vi "executeOffensivePlay.vi"(8 "error in (no error)":errorcluster, 11 "Game in":refnum<class "Game.lvclass">) -> (0 "error out":errorcluster, 3 "Game out":refnum<class "Game.lvclass">)   [LabVIEW 2023, in "Game.lvclass"]
uses:
  Game.lvclass
  Utilities_class/Utilities.lvclass
  Team_class/OffensivePlay.ctl
  Game.lvclass/Game.ctl
  Team_class/Team.lvclass/Team.ctl
  Playbook_class/Playbook.lvclass/Playbook.ctl
  TestPlay_class/TestPlay.lvclass/TestPlay.ctl
  EnemyPossessionAtOurFieldPlay_class/EnemyPossessionAtOurFieldPlay.lvclass/EnemyPossessionAtOurFieldPlay.ctl
  PreparePassPlay_class/PreparePassPlay.lvclass/PreparePassPlay.ctl
  PrepareDoublePassPlay_class/PrepareDoublePassPlay.lvclass/PrepareDoublePassPlay.ctl
  PrepareRollToPassPlay_class/PrepareRollToPassPlay.lvclass/PrepareRollToPassPlay.ctl
  TableWithStrikerPlay_class/TableWithStrikerPlay.lvclass/TableWithStrikerPlay.ctl
  TableWith2ndStrikerPlay_class/TableWith2ndStrikerPlay.lvclass/TableWith2ndStrikerPlay.ctl
  DirectEnemyPlay_class/DirectEnemyPlay.lvclass/DirectEnemyPlay.ctl
  HaltPlay_class/HaltPlay.lvclass/HaltPlay.ctl
  IndirectEnemyPlay_class/IndirectEnemyPlay.lvclass/IndirectEnemyPlay.ctl
  StopOffensivePlay_class/StopOffensivePlay.lvclass/StopOffensivePlay.ctl
  BallOutOfFieldPlay_class/BallOutOfFieldPlay.lvclass/BallOutOfFieldPlay.ctl
  EnemyPossessionAtEnemyFieldPlay_class/EnemyPossessionAtEnemyFieldPlay.lvclass/EnemyPossessionAtEnemyFieldPlay.ctl
  NormalGamePlay_class/NormalGamePlay.lvclass/NormalGamePlay.ctl
  PrepareKickoffAllyPlay_class/PrepareKickoffAllyPlay.lvclass/PrepareKickoffAllyPlay.ctl
  PreparePenaltyAllyPlay_class/PreparePenaltyAllyPlay.lvclass/PreparePenaltyAllyPlay.ctl
  PreparePenaltyEnemyPlay_class/PreparePenaltyEnemyPlay.lvclass/PreparePenaltyEnemyPlay.ctl
  PrepareKickoffEnemyPlay_class/PrepareKickoffEnemyPlay.lvclass/PrepareKickoffEnemyPlay.ctl
  KickPenaltyAllyPlay_class/KickPenaltyAllyPlay.lvclass/KickPenaltyAllyPlay.ctl
  Robot_class/Robot.lvclass/Robot.ctl
  PreparePassReceiverRole_class/PreparePassReceiverEnum.ctl
  Robot_class/Read role.vi
  Playbook_class/Read offensive_plays.vi
  TestPlay_class/Read Roles.vi
  EnemyPossessionAtOurFieldPlay_class/Read Roles.vi
  PreparePassPlay_class/Read Roles.vi
  PrepareDoublePassPlay_class/Read Roles.vi
  PrepareRollToPassPlay_class/Read Roles.vi
  TableWithStrikerPlay_class/Read Roles.vi
  TableWith2ndStrikerPlay_class/Read Roles.vi
  DirectEnemyPlay_class/Read Roles.vi
  HaltPlay_class/Read Roles.vi
  IndirectEnemyPlay_class/Read Roles.vi
  StopOffensivePlay_class/Read Roles.vi
  BallOutOfFieldPlay_class/Read Roles.vi
  EnemyPossessionAtEnemyFieldPlay_class/Read Roles.vi
  NormalGamePlay_class/Read Roles.vi
  PrepareKickoffAllyPlay_class/Read Roles.vi
  PreparePenaltyAllyPlay_class/Read Roles.vi
  Robot_class/Read id.vi
  PreparePenaltyEnemyPlay_class/Read roles.vi
  PrepareKickoffEnemyPlay_class/Read Roles.vi
  KickPenaltyAllyPlay_class/Read Roles.vi
  Read OffensiveTeam.vi
  Team_class/Read RobotRef.vi
  Team_class/Read OffensivePlay.vi
  Team_class/Write RobotRef.vi
  Team_class/Write OffensivePlay Finished.vi
  Write OffensiveTeam.vi
  Ally_class/Ally.lvclass
  C:/Users/roboi/Downloads/VSS_AI-Larc2023/Team_class/Team.lvclass
  Playbook_class/Playbook.lvclass
  Robot_class/Robot.lvclass
  Play_class/Play.lvclass
  TestPlay_class/TestPlay.lvclass
  EnemyPossessionAtEnemyFieldPlay_class/EnemyPossessionAtEnemyFieldPlay.lvclass
  EnemyPossessionAtOurFieldPlay_class/EnemyPossessionAtOurFieldPlay.lvclass
  NormalGamePlay_class/NormalGamePlay.lvclass
  IndirectEnemyPlay_class/IndirectEnemyPlay.lvclass
  PrepareKickoffAllyPlay_class/PrepareKickoffAllyPlay.lvclass
  PrepareKickoffEnemyPlay_class/PrepareKickoffEnemyPlay.lvclass
  KickPenaltyAllyPlay_class/KickPenaltyAllyPlay.lvclass
  PreparePenaltyAllyPlay_class/PreparePenaltyAllyPlay.lvclass
  DirectEnemyPlay_class/DirectEnemyPlay.lvclass
  PreparePenaltyEnemyPlay_class/PreparePenaltyEnemyPlay.lvclass
  BallOutOfFieldPlay_class/BallOutOfFieldPlay.lvclass
  StopOffensivePlay_class/StopOffensivePlay.lvclass
  PassPlay_class/PassPlay.lvclass
  DirectKickPlay_class/DirectKickPlay.lvclass
  HaltPlay_class/HaltPlay.lvclass
  PreparePassPlay_class/PreparePassPlay.lvclass
  PassToStriker_class/PassToStriker.lvclass
  PassTo2ndStriker_class/PassTo2ndStriker.lvclass
  SimplePass_class/SimplePass.lvclass
  PrepareRollToPassPlay_class/PrepareRollToPassPlay.lvclass
  PrepareDoublePassPlay_class/PrepareDoublePassPlay.lvclass
  TableWith2ndStrikerPlay_class/TableWith2ndStrikerPlay.lvclass
  TableWithStrikerPlay_class/TableWithStrikerPlay.lvclass
  TestRole_class/TestRole.lvclass
  Role_class/Role.lvclass
  ShootRole_class/ShootRole.lvclass
  MarkerRole_class/MarkerRole.lvclass
  PreparePassReceiverRole_class/PreparePassReceiverRole.lvclass
  AttackerStopRole_class/AttackerStopRole.lvclass
  PrepareRollToPassReceiverRole_class/PrepareRollToPassReceiverRole.lvclass
  PrepareRollToPassRollerRole_class/PrepareRollToPassRollerRole.lvclass
  PassKickerRole_class/PassKickerRole.lvclass
  PassReceiverRole_class/PassReceiverRole.lvclass
  PassObserverRole_class/PassObserverRole.lvclass
  TableFinalizerRole_class/TableFinalizerRole.lvclass
  TablerRole_class/TablerRole.lvclass
  AttackerBlockRole_class/AttackerBlockRole.lvclass
  HaltRole_class/HaltRole.lvclass
  BallOutOfFieldRole_class/BallOutOfFieldRole.lvclass
  FollowAttackerRole_class/FollowAttackerRole.lvclass
  AttackerAimGoalRole_class/AttackerAimGoalRole.lvclass
  PenaltyDefenseRole_class/PenaltyDefenseRole.lvclass
  SimplePassRollRole_class/SimplePassRollRole.lvclass
  SimplePassReceiverRole_class/SimplePassReceiverRole.lvclass
  PenaltyAttackerRole_class/PenaltyAttackerRole.lvclass
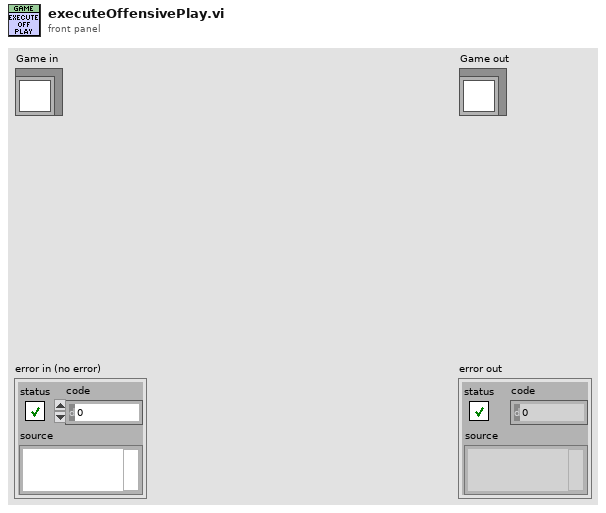
[diagram p1: front panel]
types:
  T1 = typedef "OffensivePlay.ctl" = enum16{"TableWithStriker", "TableWith2ndStrikerPlay", "PrepareDoublePass", "PrepareRollToPass", "SimplePass", "PreparePass", "PassToStriker", "BallOutOfField", "PassTo2ndStriker", "StopOffensive", "Prepare Penalty Enemy", "EnemyPossessionAtEnemyField", "EnemyPossesionAtOurField", "TestPlay", "PreparePenaltyAlly", "KickPenaltyAlly", "PrepareKickoffAlly", "PrepareKickoffEnemy", "IndirectEnemy", "DirectEnemy", "NormalGame", "DirectKick", "Pass", "Halt", "Timeout", "PassPlay", "PenaltyEnemy"}
  T2 = typedef "PreparePassReceiverEnum.ctl" = enum16{"2ndStrikerDPass", "2ndStriker", "Striker"}
  T3 = typedef "offensive_plays.ctl" = cluster{"Play":refnum<class "Play.lvclass">, "TestPlay":refnum<class "TestPlay.lvclass">, "EnemyPossessionAtEnemyFieldPlay":refnum<class "EnemyPossessionAtEnemyFieldPlay.lvclass">, "EnemyPossessionAtOurFieldPlay":refnum<class "EnemyPossessionAtOurFieldPlay.lvclass">, "NormalGamePlay":refnum<class "NormalGamePlay.lvclass">, "IndirectEnemyPlay":refnum<class "IndirectEnemyPlay.lvclass">, "PrepareKickoffAllyPlay":refnum<class "PrepareKickoffAllyPlay.lvclass">, "PrepareKickoffEnemyPlay":refnum<class "PrepareKickoffEnemyPlay.lvclass">, "KickPenaltyAllyPlay":refnum<class "KickPenaltyAllyPlay.lvclass">, "PreparePenaltyAllyPlay":refnum<class "PreparePenaltyAllyPlay.lvclass">, "DirectEnemyPlay":refnum<class "DirectEnemyPlay.lvclass">, "PreparePenaltyEnemyPlay":refnum<class "PreparePenaltyEnemyPlay.lvclass">, "BallOutOfFieldPlay":refnum<class "BallOutOfFieldPlay.lvclass">, "StopOffensivePlay":refnum<class "StopOffensivePlay.lvclass">, "PassPlay":refnum<class "PassPlay.lvclass">, "DirectKickPlay":refnum<class "DirectKickPlay.lvclass">, "HaltPlay":refnum<class "HaltPlay.lvclass">, "PreparePassPlay":refnum<class "PreparePassPlay.lvclass">, "PassToStrikerPlay":refnum<class "PassToStriker.lvclass">, "PassTo2ndStrikerPlay":refnum<class "PassTo2ndStriker.lvclass">, "SimplePassPlay":refnum<class "SimplePass.lvclass">, "PrepareRollToPassPlay":refnum<class "PrepareRollToPassPlay.lvclass">, "PrepareDoublePassPlay":refnum<class "PrepareDoublePassPlay.lvclass">, "TableWith2ndStrikerPlay":refnum<class "TableWith2ndStrikerPlay.lvclass">, "TableWithStrikerPlay":refnum<class "TableWithStrikerPlay.lvclass">}
  T4 = typedef "roles.ctl" = enum16{"BallChallengerAttackerVSS", "NormalAttackerVSS", "AttackerAimGoalVSS", "DefenderAreaVSS", "KeeperVSS", "Tabler", "TableFinalizer", "PrepareRollToPassRoller", "PrepareRollToPassReceiver", "SimplePassRoll", "SimplePassRollReceiver", "PenaltyDefense", "PreparePassReceiver 2", "PreparePassReceiver 1", "PassObserver", "Timeout", "Goto", "ZigZag", "None", "BallOutOfField", "DefenderArea", "Duelist", "AttackerStop", "FollowAttacker", "KeeperRole", "KickPenalty", "AttackerAimGoal", "AttackerBlock", "Marker", "Halt", "Shoot", "PassKicker", "PassReceiver", "TestRole", "PenaltyAttacker"}
  T5 = cluster{"TestRole 1":refnum<class "TestRole.lvclass">, "Role":refnum<class "Role.lvclass">, "TestRole 2":refnum<class "TestRole.lvclass">, "TestRole 3":refnum<class "TestRole.lvclass">}
  T6 = cluster{"ShootRole":refnum<class "ShootRole.lvclass">, "MarkerRole":refnum<class "MarkerRole.lvclass">}
  T7 = cluster{"PreparePassReceiverRole 1":refnum<class "PreparePassReceiverRole.lvclass">, "AttackerStopRole":refnum<class "AttackerStopRole.lvclass">, "PreparePassReceiverRole 2":refnum<class "PreparePassReceiverRole.lvclass">}
  T8 = cluster{"AttackerStopRole":refnum<class "AttackerStopRole.lvclass">, "PreparePassReceiverRole 1":refnum<class "PreparePassReceiverRole.lvclass">, "PreparePassReceiverRole 2":refnum<class "PreparePassReceiverRole.lvclass">}
  T9 = cluster{"PreparePassReceiverRole 1":refnum<class "PreparePassReceiverRole.lvclass">, "PreparePassReceiverRole 2":refnum<class "PreparePassReceiverRole.lvclass">, "PrepareRollToPassReceiverRole":refnum<class "PrepareRollToPassReceiverRole.lvclass">, "PrepareRollToPassRollerRole":refnum<class "PrepareRollToPassRollerRole.lvclass">}
  T10 = cluster{"PassKickerRole":refnum<class "PassKickerRole.lvclass">, "PassReceiverRole":refnum<class "PassReceiverRole.lvclass">, "PassObserverRole":refnum<class "PassObserverRole.lvclass">}
  T11 = cluster{"TableFinalizerRole":refnum<class "TableFinalizerRole.lvclass">, "TablerRole":refnum<class "TablerRole.lvclass">, "PassObserverRole":refnum<class "PassObserverRole.lvclass">}
  T12 = cluster{"AttackerBlockRole":refnum<class "AttackerBlockRole.lvclass">, "MarkerRole":refnum<class "MarkerRole.lvclass">}
  T13 = cluster{"HaltRole 1":refnum<class "HaltRole.lvclass">, "HaltRole 2":refnum<class "HaltRole.lvclass">, "HaltRole 3":refnum<class "HaltRole.lvclass">, "HaltRole 4":refnum<class "HaltRole.lvclass">, "HaltRole 5":refnum<class "HaltRole.lvclass">, "HaltRole 6":refnum<class "HaltRole.lvclass">}
  T14 = cluster{"MarkerRole":refnum<class "MarkerRole.lvclass">, "AttackerStopRole":refnum<class "AttackerStopRole.lvclass">}
  T15 = cluster{"BallOutOfFieldRole":refnum<class "BallOutOfFieldRole.lvclass">, "FollowAttackerRole":refnum<class "FollowAttackerRole.lvclass">}
  T16 = cluster{"ShootRole":refnum<class "ShootRole.lvclass">, "FollowAttackerRole":refnum<class "FollowAttackerRole.lvclass">}
  T17 = cluster{"AttackerAimGoalRole":refnum<class "AttackerAimGoalRole.lvclass">, "FollowAttackerRole":refnum<class "FollowAttackerRole.lvclass">}
  T18 = cluster{"AttackerAimGoalRole":refnum<class "AttackerAimGoalRole.lvclass">}
  T19 = cluster{"PenaltyDefenseRole 1":refnum<class "PenaltyDefenseRole.lvclass">, "PenaltyDefenseRole 2":refnum<class "PenaltyDefenseRole.lvclass">, "PenaltyDefenseRole 3":refnum<class "PenaltyDefenseRole.lvclass">, "PenaltyDefenseRole 4":refnum<class "PenaltyDefenseRole.lvclass">, "PenaltyDefenseRole 5":refnum<class "PenaltyDefenseRole.lvclass">}
  T20 = cluster{"SimplePassRollRole":refnum<class "SimplePassRollRole.lvclass">, "SimplePassReceiverRole":refnum<class "SimplePassReceiverRole.lvclass">}
  T21 = cluster{"AttackerBlockRole":refnum<class "AttackerBlockRole.lvclass">, "FollowAttackerRole":refnum<class "FollowAttackerRole.lvclass">}
  T22 = cluster{"PenaltyAttackerRole":refnum<class "PenaltyAttackerRole.lvclass">}
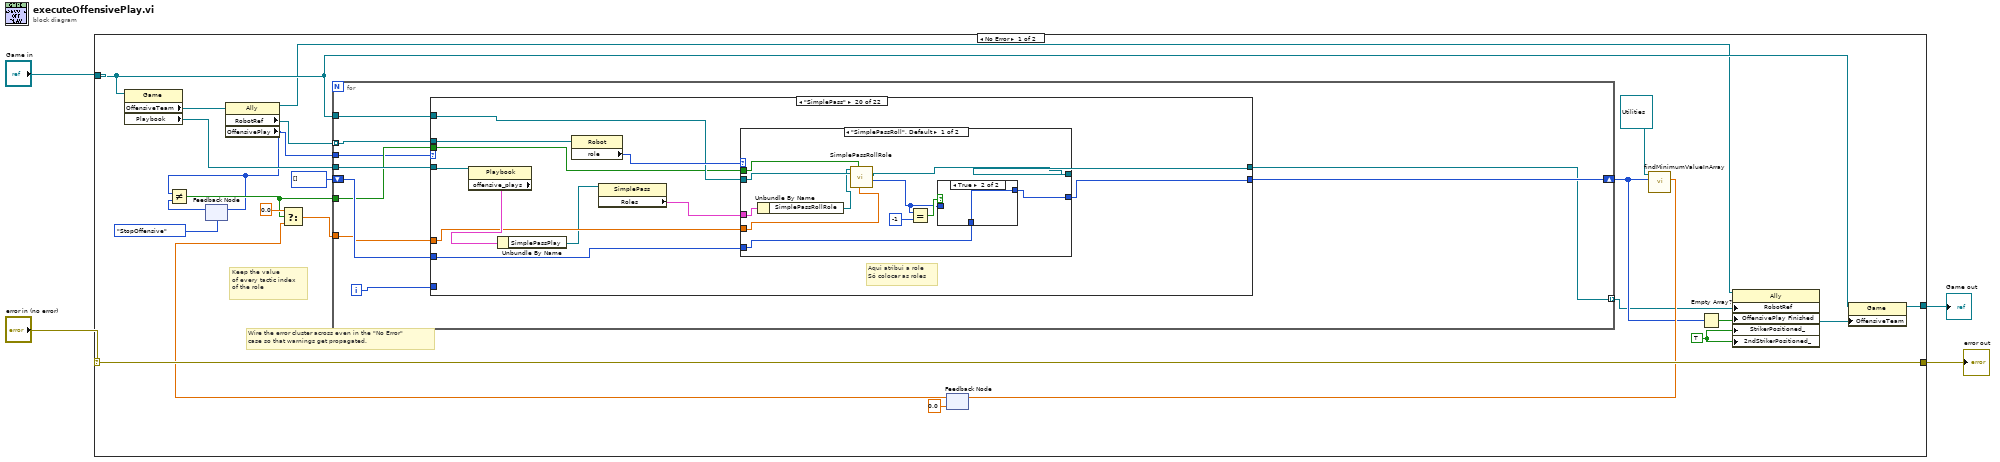
[diagram p0: block diagram]
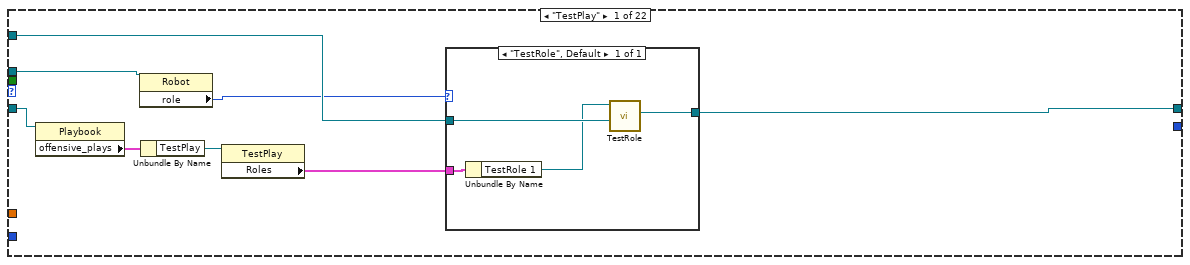
[diagram p2: hidden frame]
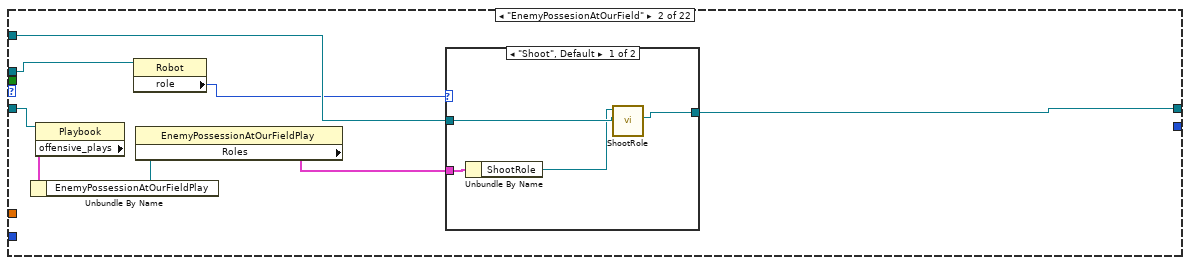
[diagram p3: hidden frame]
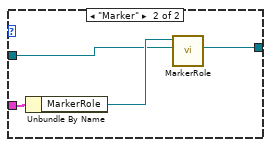
[diagram p4: hidden frame]
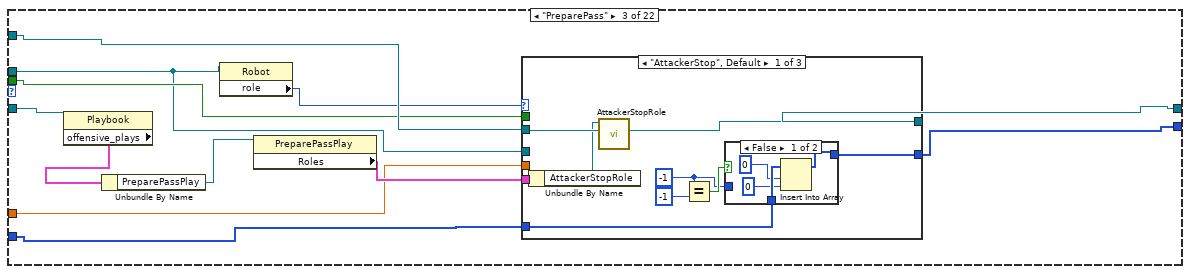
[diagram p5: hidden frame]
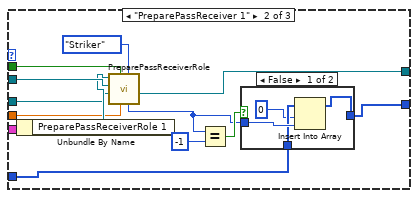
[diagram p7: hidden frame]
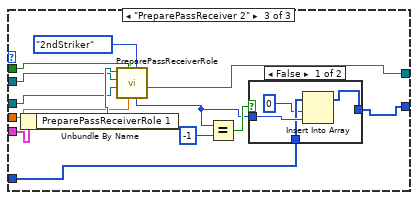
[diagram p9: hidden frame]
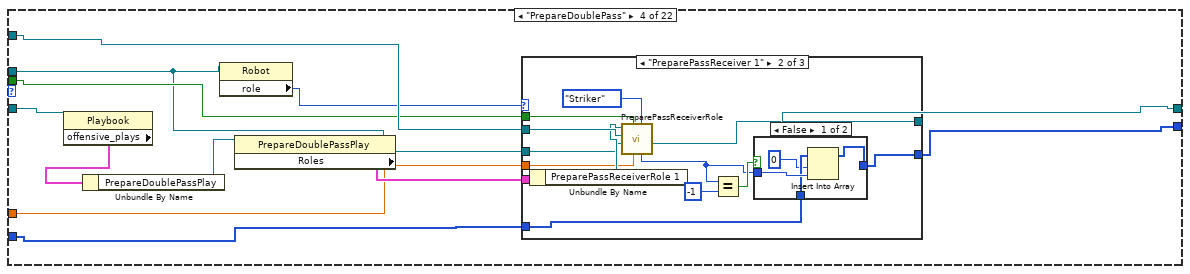
[diagram p11: hidden frame]
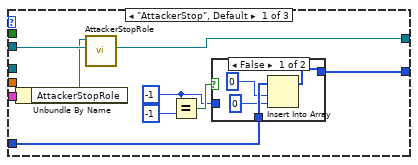
[diagram p12: hidden frame]
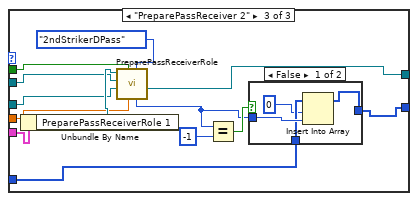
[diagram p15: hidden frame]
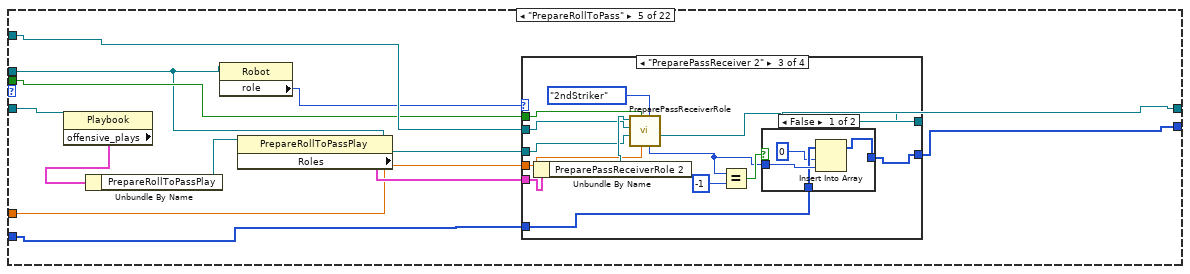
[diagram p17: hidden frame]
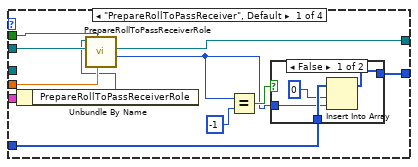
[diagram p18: hidden frame]
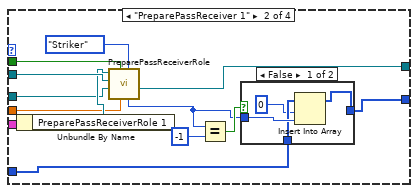
[diagram p20: hidden frame]
diagram:
  n1 = case shown="No Error" "error in (no error)" {
    selector: "error in (no error)" -> [w27 w748]
    tunnel: [w27 w748] -> w1
    tunnel: [w23 w747] -> w2
    tunnel: "Game in" -> [w8 w747]
    frame No Error {
      w10 = TRUE
      # "Keep the value\nof every tactic index\nof the role"
      # "Wire the error cluster across even in the \"No Error\"\ncase so that warnings get propagated."
      n2 = property class="Game"(reference=w8) -> ("OffensiveTeam"=w26:refnum<class "Ally.lvclass">, "Playbook"=w24:refnum<class "Playbook.lvclass">)  [unwired: 1 in, 2 out]
      n3 = feedback #1(OffensivePlay."StopOffensive" ("OffensivePlay")) -> (w18:T1)
      n4 = property class="Ally"(reference=w26) -> (reference out=w7:refnum<class "Ally.lvclass">, "RobotRef"=w25:refnum<class "Robot.lvclass">[], "OffensivePlay"=w5:T1)  [unwired: 1 in, 1 out]
      n5 = Not Equal?(x=w5, y=w18) -> (x != y?=w14:bool)
      n6 = feedback-in #1(w5) -> ()
      n7 = feedback #2(0.0 ("minimum")) -> (w16:dbl)
      n8 = Select(t=0.0, s=w14, f=w16) -> (s? t:f=w9:dbl)
      n9 = for {
        tunnel: w25 -> [w32] mode=indexing
        tunnel: w24 -> [w37]
        tunnel: w8 -> [w36]
        shift-right: [w35] -> w12
        shift-left: i32[] [] -> [w34]
        tunnel: w14 -> [w33]
        tunnel: w9 -> [w31]
        tunnel: [w29] -> w6 mode=indexing
        tunnel: w5 -> [w28]
        i -> [w30]
        n10 = case shown="\"SimplePass\"" w28 {
          tunnel: w37 -> [w45 w57 w70 w132 w194 w277 w337 w397 w457 w517 w533 w545 w561 w577 w593 w609 w625 w641 w654 w680 w726 w742]
          tunnel: w36 -> [w41 w53 w72 w134 w196 w279 w340 w400 w460 w513 w529 w541 w557 w573 w589 w605 w621 w637 w650 w682 w722 w738]
          tunnel: [w40 w52 w75 w137 w199 w274 w336 w396 w456 w512 w528 w540 w556 w572 w588 w604 w620 w636 w648 w684 w721 w737] -> w29
          tunnel: w31 -> [_ _ w68 w130 w192 w270 w330 w390 w450 _ _ _ _ _ _ _ _ _ _ w679 _ _]
          tunnel: [_ _ w74 w136 w198 w273 w335 w395 w455 _ _ _ _ _ _ _ _ _ _ w683 _ _] -> w35
          tunnel: w34 -> [_ _ w73 w135 w197 w272 w334 w394 w454 _ _ _ _ _ _ _ _ _ _ w678 _ _]
          tunnel: w33 -> [_ _ w71 w133 w195 w271 w338 w398 w458 _ _ _ _ _ _ _ _ _ _ w681 _ _]
          tunnel: w32 -> [w39 w51 w67 w129 w191 w278 w339 w399 w459 w511 w527 w539 w554 w571 w587 w603 w619 w635 w649 w677 w720 w736]
          tunnel: w30 -> [_ _ _ _ _ _ _ _ _ _ _ _ _ _ _ _ _ _ w646 _ _ _]
          frame "TestPlay" {
            n11 = property class="Playbook"(reference=w45) -> ("offensive_plays"=w44:T3)  [unwired: 1 in, 2 out]
            n12 = property class="Robot"(reference=w39) -> ("role"=w38:T4)  [unwired: 1 in, 2 out]
            n13 = Unbundle By Name(w44) -> ("TestPlay"=w43:refnum<class "TestPlay.lvclass">)
            n14 = property class="TestPlay"(reference=w43) -> ("Roles"=w42:T5)  [unwired: 1 in, 2 out]
            n15 = case shown="\"TestRole\", Default" w38 {
              tunnel: w42 -> [w49]
              tunnel: w41 -> [w48]
              tunnel: [w47] -> w40
              frame "TestRole", Default {
                n16 = Unbundle By Name(w49) -> ("TestRole 1"=w46:refnum<class "TestRole.lvclass">)
                n17 = call-dynamic "TestRole.vi"("Game in"=w48, "TestRole in"=w46) -> ("Robot out"=w47:refnum<class "Robot.lvclass">)  [unwired: 6 in, 3 out]
              }
            }
          }
          frame "EnemyPossesionAtOurField" {
            n18 = property class="Playbook"(reference=w57) -> ("offensive_plays"=w56:T3)  [unwired: 1 in, 2 out]
            n19 = Unbundle By Name(w56) -> ("EnemyPossessionAtOurFieldPlay"=w55:refnum<class "EnemyPossessionAtOurFieldPlay.lvclass">)
            n20 = property class="Robot"(reference=w51) -> ("role"=w50:T4)  [unwired: 1 in, 2 out]
            n21 = property class="EnemyPossessionAtOurFieldPlay"(reference=w55) -> ("Roles"=w54:T6)  [unwired: 1 in, 2 out]
            n22 = case shown="\"Shoot\", Default" w50 {
              tunnel: w54 -> [w61 w65]
              tunnel: w53 -> [w60 w63]
              tunnel: [w58 w62] -> w52
              frame "Shoot", Default {
                n23 = Unbundle By Name(w61) -> ("ShootRole"=w59:refnum<class "ShootRole.lvclass">)
                n24 = call-dynamic "ShootRole.vi"("Game in"=w60, "ShootRole in"=w59) -> ("Robot out"=w58:refnum<class "Robot.lvclass">)  [unwired: 6 in, 3 out]
              }
              frame "Marker" {
                n25 = Unbundle By Name(w65) -> ("MarkerRole"=w64:refnum<class "MarkerRole.lvclass">)
                n26 = call-dynamic "MarkerRole.vi"("Game in"=w63, "MarkerRole in"=w64) -> ("Robot out"=w62:refnum<class "Robot.lvclass">)  [unwired: 6 in, 3 out]
              }
            }
          }
          frame "PreparePass" {
            n27 = property class="Playbook"(reference=w70) -> ("offensive_plays"=w69:T3)  [unwired: 1 in, 2 out]
            n28 = Unbundle By Name(w69) -> ("PreparePassPlay"=w76:refnum<class "PreparePassPlay.lvclass">)
            n29 = property class="Robot"(reference=w67) -> ("role"=w66:T4)  [unwired: 1 in, 2 out]
            n30 = property class="PreparePassPlay"(reference=w76) -> ("Roles"=w77:T7)  [unwired: 1 in, 2 out]
            n31 = case shown="\"AttackerStop\", Default" w66 {
              tunnel: w77 -> [w86 w101 w118]
              tunnel: w72 -> [w81 w102 w113]
              tunnel: [w85 w97 w115] -> w75
              tunnel: [w83 w96 w116] -> w74
              tunnel: w73 -> [w82 w99 w117]
              tunnel: w71 -> [_ w95 w114]
              tunnel: w68 -> [_ w94 w111]
              tunnel: w67 -> [_ w93 w112]
              frame "AttackerStop", Default {
                w78 = -1 ("x")
                n32 = Unbundle By Name(w86) -> ("AttackerStopRole"=w80:refnum<class "AttackerStopRole.lvclass">)
                n33 = call-dynamic "AttackerStopRole.vi"("Game in"=w81, "AttackerStopRole in"=w80) -> ("Robot out"=w85:refnum<class "Robot.lvclass">)  [unwired: 6 in, 3 out]
                n34 = Equal?(x=w78, y=-1) -> (x = y?=w84:bool)
                n35 = case shown="False" w84 {
                  tunnel: w82 -> [w90 w91]
                  tunnel: [w89 w91] -> w83
                  tunnel: w78 -> [_ _]
                  frame False {
                    n36 = Insert Into Array(array=w90, index=0, new element=0 ("new element/subarray")) -> (w89:i32[])
                  }
                  frame True {
                  }
                }
              }
              frame "PreparePassReceiver 1" {
                n37 = Unbundle By Name(w101) -> ("PreparePassReceiverRole 1"=w100:refnum<class "PreparePassReceiverRole.lvclass">)
                n38 = call "PreparePassReceiverRole.vi"("Striker/2ndStriker"=PreparePassReceiverEnum."Striker", "Tactic index in"=w94, "first call"=w95, "RobotRef"=w93, "Game in"=w102, "PreparePassReceiverRole in"=w100) -> ("Robot out"=w97:refnum<class "Robot.lvclass">, "tactic index"=w98:i32)  [unwired: 1 in, 3 out]
                n39 = Equal?(x=w98, y=-1) -> (x = y?=w103:bool)
                n40 = case shown="False" w103 {
                  tunnel: w98 -> [w108 _]
                  tunnel: w99 -> [w107 w109]
                  tunnel: [w105 w109] -> w96
                  frame False {
                    n41 = Insert Into Array(array=w107, index=0, new element=w108) -> (w105:i32[])
                  }
                  frame True {
                  }
                }
              }
              frame "PreparePassReceiver 2" {
                n42 = Unbundle By Name(w118) -> ("PreparePassReceiverRole 1"=w120:refnum<class "PreparePassReceiverRole.lvclass">)
                n43 = call "PreparePassReceiverRole.vi"("Striker/2ndStriker"=PreparePassReceiverEnum."2ndStriker", "Tactic index in"=w111, "first call"=w114, "RobotRef"=w112, "Game in"=w113, "PreparePassReceiverRole in"=w120) -> ("Robot out"=w115:refnum<class "Robot.lvclass">, "tactic index"=w119:i32)  [unwired: 1 in, 3 out]
                n44 = Equal?(x=w119, y=-1) -> (x = y?=w121:bool)
                n45 = case shown="False" w121 {
                  tunnel: w119 -> [w126 _]
                  tunnel: w117 -> [w125 w127]
                  tunnel: [w123 w127] -> w116
                  frame False {
                    n46 = Insert Into Array(array=w125, index=0, new element=w126) -> (w123:i32[])
                  }
                  frame True {
                  }
                }
              }
            }
          }
          frame "PrepareDoublePass" {
            n47 = property class="Playbook"(reference=w132) -> ("offensive_plays"=w131:T3)  [unwired: 1 in, 2 out]
            n48 = Unbundle By Name(w131) -> ("PrepareDoublePassPlay"=w138:refnum<class "PrepareDoublePassPlay.lvclass">)
            n49 = property class="Robot"(reference=w129) -> ("role"=w128:T4)  [unwired: 1 in, 2 out]
            n50 = property class="PrepareDoublePassPlay"(reference=w138) -> ("Roles"=w139:T8)  [unwired: 1 in, 2 out]
            n51 = case shown="\"PreparePassReceiver 1\"" w128 {
              tunnel: w139 -> [w148 w163 w180]
              tunnel: w134 -> [w143 w164 w175]
              tunnel: [w147 w159 w177] -> w137
              tunnel: [w145 w158 w178] -> w136
              tunnel: w135 -> [w144 w161 w179]
              tunnel: w133 -> [_ w157 w176]
              tunnel: w130 -> [_ w156 w173]
              tunnel: w129 -> [_ w155 w174]
              frame "AttackerStop", Default {
                w140 = -1 ("x")
                n52 = Unbundle By Name(w148) -> ("AttackerStopRole"=w142:refnum<class "AttackerStopRole.lvclass">)
                n53 = call-dynamic "AttackerStopRole.vi"("Game in"=w143, "AttackerStopRole in"=w142) -> ("Robot out"=w147:refnum<class "Robot.lvclass">)  [unwired: 6 in, 3 out]
                n54 = Equal?(x=w140, y=-1) -> (x = y?=w146:bool)
                n55 = case shown="False" w146 {
                  tunnel: w144 -> [w152 w153]
                  tunnel: [w151 w153] -> w145
                  tunnel: w140 -> [_ _]
                  frame False {
                    n56 = Insert Into Array(array=w152, index=0, new element=0 ("new element/subarray")) -> (w151:i32[])
                  }
                  frame True {
                  }
                }
              }
              frame "PreparePassReceiver 1" {
                n57 = Unbundle By Name(w163) -> ("PreparePassReceiverRole 1"=w162:refnum<class "PreparePassReceiverRole.lvclass">)
                n58 = call "PreparePassReceiverRole.vi"("Striker/2ndStriker"=PreparePassReceiverEnum."Striker", "Tactic index in"=w156, "first call"=w157, "RobotRef"=w155, "Game in"=w164, "PreparePassReceiverRole in"=w162) -> ("Robot out"=w159:refnum<class "Robot.lvclass">, "tactic index"=w160:i32)  [unwired: 1 in, 3 out]
                n59 = Equal?(x=w160, y=-1) -> (x = y?=w165:bool)
                n60 = case shown="False" w165 {
                  tunnel: w160 -> [w170 _]
                  tunnel: w161 -> [w169 w171]
                  tunnel: [w167 w171] -> w158
                  frame False {
                    n61 = Insert Into Array(array=w169, index=0, new element=w170) -> (w167:i32[])
                  }
                  frame True {
                  }
                }
              }
              frame "PreparePassReceiver 2" {
                n62 = Unbundle By Name(w180) -> ("PreparePassReceiverRole 1"=w182:refnum<class "PreparePassReceiverRole.lvclass">)
                n63 = call "PreparePassReceiverRole.vi"("Striker/2ndStriker"=PreparePassReceiverEnum."2ndStrikerDPass" ("Enum"), "Tactic index in"=w173, "first call"=w176, "RobotRef"=w174, "Game in"=w175, "PreparePassReceiverRole in"=w182) -> ("Robot out"=w177:refnum<class "Robot.lvclass">, "tactic index"=w181:i32)  [unwired: 1 in, 3 out]
                n64 = Equal?(x=w181, y=-1) -> (x = y?=w183:bool)
                n65 = case shown="False" w183 {
                  tunnel: w181 -> [w188 _]
                  tunnel: w179 -> [w187 w189]
                  tunnel: [w185 w189] -> w178
                  frame False {
                    n66 = Insert Into Array(array=w187, index=0, new element=w188) -> (w185:i32[])
                  }
                  frame True {
                  }
                }
              }
            }
          }
          frame "PrepareRollToPass" {
            n67 = property class="Playbook"(reference=w194) -> ("offensive_plays"=w193:T3)  [unwired: 1 in, 2 out]
            n68 = Unbundle By Name(w193) -> ("PrepareRollToPassPlay"=w200:refnum<class "PrepareRollToPassPlay.lvclass">)
            n69 = property class="Robot"(reference=w191) -> ("role"=w190:T4)  [unwired: 1 in, 2 out]
            n70 = property class="PrepareRollToPassPlay"(reference=w200) -> ("Roles"=w201:T9)  [unwired: 1 in, 2 out]
            n71 = case shown="\"PreparePassReceiver 2\"" w190 {
              tunnel: w201 -> [w212 w227 w244 w262]
              tunnel: w196 -> [w207 w228 w239 w254]
              tunnel: [w211 w223 w241 w255] -> w199
              tunnel: [w209 w222 w242 w260] -> w198
              tunnel: w197 -> [w208 w225 w243 w261]
              tunnel: w195 -> [w205 w221 w240 w258]
              tunnel: w192 -> [w204 w220 w237 w257]
              tunnel: w191 -> [_ w219 w238 _]
              frame "PrepareRollToPassReceiver", Default {
                n72 = Unbundle By Name(w212) -> ("PrepareRollToPassReceiverRole"=w202:refnum<class "PrepareRollToPassReceiverRole.lvclass">)
                n73 = call "PrepareRollToPassReceiverRole.vi"("Tactic index in"=w204, "first call"=w205, "Game in"=w207, "PrepareRollToPassReceiverRole in"=w202) -> ("tactic index"=w203:i32, "Robot out"=w211:refnum<class "Robot.lvclass">)  [unwired: 4 in, 2 out]
                n74 = Equal?(x=w203, y=-1) -> (x = y?=w210:bool)
                n75 = case shown="False" w210 {
                  tunnel: w208 -> [w216 w217]
                  tunnel: [w215 w217] -> w209
                  tunnel: w203 -> [w213 _]
                  frame False {
                    n76 = Insert Into Array(array=w216, index=0 ("new element/subarray"), new element=w213) -> (w215:i32[])
                  }
                  frame True {
                  }
                }
              }
              frame "PreparePassReceiver 1" {
                n77 = Unbundle By Name(w227) -> ("PreparePassReceiverRole 1"=w226:refnum<class "PreparePassReceiverRole.lvclass">)
                n78 = call "PreparePassReceiverRole.vi"("Striker/2ndStriker"=PreparePassReceiverEnum."Striker", "Tactic index in"=w220, "first call"=w221, "RobotRef"=w219, "Game in"=w228, "PreparePassReceiverRole in"=w226) -> ("Robot out"=w223:refnum<class "Robot.lvclass">, "tactic index"=w224:i32)  [unwired: 1 in, 3 out]
                n79 = Equal?(x=w224, y=-1) -> (x = y?=w229:bool)
                n80 = case shown="False" w229 {
                  tunnel: w224 -> [w234 _]
                  tunnel: w225 -> [w233 w235]
                  tunnel: [w231 w235] -> w222
                  frame False {
                    n81 = Insert Into Array(array=w233, index=0, new element=w234) -> (w231:i32[])
                  }
                  frame True {
                  }
                }
              }
              frame "PreparePassReceiver 2" {
                n82 = Unbundle By Name(w244) -> ("PreparePassReceiverRole 2"=w246:refnum<class "PreparePassReceiverRole.lvclass">)
                n83 = call "PreparePassReceiverRole.vi"("Striker/2ndStriker"=PreparePassReceiverEnum."2ndStriker", "Tactic index in"=w237, "first call"=w240, "RobotRef"=w238, "Game in"=w239, "PreparePassReceiverRole in"=w246) -> ("Robot out"=w241:refnum<class "Robot.lvclass">, "tactic index"=w245:i32)  [unwired: 1 in, 3 out]
                n84 = Equal?(x=w245, y=-1) -> (x = y?=w247:bool)
                n85 = case shown="False" w247 {
                  tunnel: w245 -> [w252 _]
                  tunnel: w243 -> [w251 w253]
                  tunnel: [w249 w253] -> w242
                  frame False {
                    n86 = Insert Into Array(array=w251, index=0, new element=w252) -> (w249:i32[])
                  }
                  frame True {
                  }
                }
              }
              frame "PrepareRollToPassRoller" {
                n87 = Unbundle By Name(w262) -> ("PrepareRollToPassRollerRole"=w259:refnum<class "PrepareRollToPassRollerRole.lvclass">)
                n88 = call "PrepareRollToPassRollerRole.vi"("Tactic index in"=w257, "first call"=w258, "Game in"=w254, "PrepareRollToPassRollerRole in"=w259) -> ("tactic index"=w256:i32, "Robot out"=w255:refnum<class "Robot.lvclass">)  [unwired: 4 in, 2 out]
                n89 = Equal?(x=w256, y=-1) -> (x = y?=w263:bool)
                n90 = case shown="False" w263 {
                  tunnel: w256 -> [w268 _]
                  tunnel: w261 -> [w267 w269]
                  tunnel: [w265 w269] -> w260
                  frame False {
                    n91 = Insert Into Array(array=w267, index=0, new element=w268) -> (w265:i32[])
                  }
                  frame True {
                  }
                }
              }
            }
          }
          frame "PassToStriker" {
            n92 = property class="Playbook"(reference=w277) -> ("offensive_plays"=w276:T3)  [unwired: 1 in, 2 out]
            n93 = Unbundle By Name(w276) -> ("PassToStrikerPlay"=w275:refnum<class "PassToStriker.lvclass">)
            n94 = property class="Robot"(reference=w278) -> ("role"=w281:T4)  [unwired: 1 in, 2 out]
            n95 = property class="PassToStriker"(reference=w275) -> ("Roles"=w280:T10)  [unwired: 1 in, 2 out]
            n96 = case shown="\"PassReceiver\"" w281 {
              tunnel: w280 -> [w289 w308 w324]
              tunnel: w279 -> [w290 w301 w323]
              tunnel: [w285 w307 w322] -> w274
              tunnel: [w284 w303 w317] -> w273
              tunnel: w272 -> [w287 w302 w318]
              tunnel: w271 -> [w283 w299 w315]
              tunnel: w270 -> [w282 w298 w314]
              frame "PassObserver" {
                n97 = Unbundle By Name(w289) -> ("PassObserverRole"=w288:refnum<class "PassObserverRole.lvclass">)
                n98 = call "PassObserverRole.vi"("Tactic index in"=w282, "first call"=w283, "Game in"=w290, "PassObserverRole in"=w288) -> ("tactic index"=w286:i32, "Robot"=w285:refnum<class "Robot.lvclass">)  [unwired: 5 in, 1 out]
                n99 = Equal?(x=w286, y=-1) -> (x = y?=w291:bool)
                n100 = case shown="False" w291 {
                  tunnel: w286 -> [w296 _]
                  tunnel: w287 -> [w295 w297]
                  tunnel: [w294 w297] -> w284
                  frame False {
                    n101 = Insert Into Array(array=w295, index=0, new element=w296) -> (w294:i32[])
                  }
                  frame True {
                  }
                }
              }
              frame "PassKicker", Default {
                n102 = Unbundle By Name(w308) -> ("PassKickerRole"=w300:refnum<class "PassKickerRole.lvclass">)
                n103 = call "PassKickerRole.vi"("Tactic index in"=w298, "first call"=w299, "Game in"=w301, "PassKickerRole in"=w300) -> ("tactic index"=w304:i32, "Robot out"=w307:refnum<class "Robot.lvclass">)  [unwired: 4 in, 2 out]
                n104 = Equal?(x=w304, y=-1) -> (x = y?=w305:bool)
                n105 = case shown="False" w305 {
                  tunnel: w304 -> [w312 _]
                  tunnel: w302 -> [w311 w313]
                  tunnel: [w310 w313] -> w303
                  frame False {
                    n106 = Insert Into Array(array=w311, index=0, new element=w312) -> (w310:i32[])
                  }
                  frame True {
                  }
                }
              }
              frame "PassReceiver" {
                n107 = Unbundle By Name(w324) -> ("PassReceiverRole"=w316:refnum<class "PassReceiverRole.lvclass">)
                n108 = call "PassReceiverRole.vi"("Tactic index in"=w314, "first call"=w315, "Game in"=w323, "PassReceiverRole in"=w316) -> ("tactic index"=w319:i32, "Robot out"=w322:refnum<class "Robot.lvclass">)  [unwired: 4 in, 2 out]
                n109 = Equal?(x=w319, y=-1) -> (x = y?=w321:bool)
                n110 = case shown="True" w321 {
                  tunnel: w319 -> [w328 _]
                  tunnel: w318 -> [w327 w329]
                  tunnel: [w326 w329] -> w317
                  frame False {
                    n111 = Insert Into Array(array=w327, index=0, new element=w328) -> (w326:i32[])
                  }
                  frame True {
                  }
                }
              }
            }
          }
          frame "PassTo2ndStriker" {
            n112 = property class="Playbook"(reference=w337) -> ("offensive_plays"=w333:T3)  [unwired: 1 in, 2 out]
            n113 = Unbundle By Name(w333) -> ("PassTo2ndStrikerPlay"=w331:refnum<class "PassTo2ndStriker.lvclass">)
            n114 = property class="Robot"(reference=w339) -> ("role"=w341:T4)  [unwired: 1 in, 2 out]
            n115 = property class="PassTo2ndStriker"(reference=w331) -> ("Roles"=w332:T10)  [unwired: 1 in, 2 out]
            n116 = case shown="\"PassObserver\"" w341 {
              tunnel: w332 -> [w349 w368 w384]
              tunnel: w340 -> [w350 w361 w383]
              tunnel: [w345 w367 w382] -> w336
              tunnel: [w344 w363 w377] -> w335
              tunnel: w334 -> [w347 w362 w378]
              tunnel: w338 -> [w343 w359 w375]
              tunnel: w330 -> [w342 w358 w374]
              frame "PassObserver" {
                n117 = Unbundle By Name(w349) -> ("PassObserverRole"=w348:refnum<class "PassObserverRole.lvclass">)
                n118 = call "PassObserverRole.vi"("Tactic index in"=w342, "first call"=w343, "Game in"=w350, "PassObserverRole in"=w348) -> ("tactic index"=w346:i32, "Robot"=w345:refnum<class "Robot.lvclass">)  [unwired: 5 in, 1 out]
                n119 = Equal?(x=w346, y=-1) -> (x = y?=w351:bool)
                n120 = case shown="True" w351 {
                  tunnel: w346 -> [w356 _]
                  tunnel: w347 -> [w355 w357]
                  tunnel: [w354 w357] -> w344
                  frame False {
                    n121 = Insert Into Array(array=w355, index=0, new element=w356) -> (w354:i32[])
                  }
                  frame True {
                  }
                }
              }
              frame "PassKicker", Default {
                n122 = Unbundle By Name(w368) -> ("PassKickerRole"=w360:refnum<class "PassKickerRole.lvclass">)
                n123 = call "PassKickerRole.vi"("Tactic index in"=w358, "first call"=w359, "Game in"=w361, "PassKickerRole in"=w360) -> ("tactic index"=w364:i32, "Robot out"=w367:refnum<class "Robot.lvclass">)  [unwired: 4 in, 2 out]
                n124 = Equal?(x=w364, y=-1) -> (x = y?=w365:bool)
                n125 = case shown="True" w365 {
                  tunnel: w364 -> [w372 _]
                  tunnel: w362 -> [w371 w373]
                  tunnel: [w370 w373] -> w363
                  frame False {
                    n126 = Insert Into Array(array=w371, index=0, new element=w372) -> (w370:i32[])
                  }
                  frame True {
                  }
                }
              }
              frame "PassReceiver" {
                n127 = Unbundle By Name(w384) -> ("PassReceiverRole"=w376:refnum<class "PassReceiverRole.lvclass">)
                n128 = call "PassReceiverRole.vi"("Tactic index in"=w374, "first call"=w375, "Game in"=w383, "PassReceiverRole in"=w376) -> ("tactic index"=w379:i32, "Robot out"=w382:refnum<class "Robot.lvclass">)  [unwired: 4 in, 2 out]
                n129 = Equal?(x=w379, y=-1) -> (x = y?=w381:bool)
                n130 = case shown="False" w381 {
                  tunnel: w379 -> [w388 _]
                  tunnel: w378 -> [w387 w389]
                  tunnel: [w386 w389] -> w377
                  frame False {
                    n131 = Insert Into Array(array=w387, index=0, new element=w388) -> (w386:i32[])
                  }
                  frame True {
                  }
                }
              }
            }
          }
          frame "TableWithStriker" {
            n132 = property class="Playbook"(reference=w397) -> ("offensive_plays"=w393:T3)  [unwired: 1 in, 2 out]
            n133 = Unbundle By Name(w393) -> ("TableWithStrikerPlay"=w391:refnum<class "TableWithStrikerPlay.lvclass">)
            n134 = property class="Robot"(reference=w399) -> ("role"=w401:T4)  [unwired: 1 in, 2 out]
            n135 = property class="TableWithStrikerPlay"(reference=w391) -> ("Roles"=w392:T11)  [unwired: 1 in, 2 out]
            n136 = case shown="\"TableFinalizer\", Default" w401 {
              tunnel: w392 -> [w409 w428 w444]
              tunnel: w400 -> [w410 w421 w443]
              tunnel: [w405 w427 w442] -> w396
              tunnel: [w404 w423 w437] -> w395
              tunnel: w394 -> [w407 w422 w438]
              tunnel: w398 -> [w403 w419 w435]
              tunnel: w390 -> [w402 w418 w434]
              frame "PassObserver" {
                n137 = Unbundle By Name(w409) -> ("PassObserverRole"=w408:refnum<class "PassObserverRole.lvclass">)
                n138 = call "PassObserverRole.vi"("Tactic index in"=w402, "first call"=w403, "Game in"=w410, "PassObserverRole in"=w408) -> ("tactic index"=w406:i32, "Robot"=w405:refnum<class "Robot.lvclass">)  [unwired: 5 in, 1 out]
                n139 = Equal?(x=w406, y=-1) -> (x = y?=w411:bool)
                n140 = case shown="True" w411 {
                  tunnel: w406 -> [w416 _]
                  tunnel: w407 -> [w415 w417]
                  tunnel: [w414 w417] -> w404
                  frame False {
                    n141 = Insert Into Array(array=w415, index=0, new element=w416) -> (w414:i32[])
                  }
                  frame True {
                  }
                }
              }
              frame "TableFinalizer", Default {
                n142 = Unbundle By Name(w428) -> ("TableFinalizerRole"=w420:refnum<class "TableFinalizerRole.lvclass">)
                n143 = call "TableFinalizerRole.vi"("Tactic index in"=w418, "first call"=w419, "Game in"=w421, "TableFinalizerRole in"=w420) -> ("tactic index"=w424:i32, "Robot out"=w427:refnum<class "Robot.lvclass">)  [unwired: 4 in, 2 out]
                n144 = Equal?(x=w424, y=-1) -> (x = y?=w425:bool)
                n145 = case shown="True" w425 {
                  tunnel: w424 -> [w432 _]
                  tunnel: w422 -> [w431 w433]
                  tunnel: [w430 w433] -> w423
                  frame False {
                    n146 = Insert Into Array(array=w431, index=0, new element=w432) -> (w430:i32[])
                  }
                  frame True {
                  }
                }
              }
              frame "Tabler" {
                n147 = Unbundle By Name(w444) -> ("TablerRole"=w436:refnum<class "TablerRole.lvclass">)
                n148 = call "TablerRole.vi"("Tactic index in"=w434, "first call"=w435, "Game in"=w443, "TablerRole in"=w436) -> ("tactic index"=w439:i32, "Robot out"=w442:refnum<class "Robot.lvclass">)  [unwired: 4 in, 2 out]
                n149 = Equal?(x=w439, y=-1) -> (x = y?=w441:bool)
                n150 = case shown="False" w441 {
                  tunnel: w439 -> [w448 _]
                  tunnel: w438 -> [w447 w449]
                  tunnel: [w446 w449] -> w437
                  frame False {
                    n151 = Insert Into Array(array=w447, index=0, new element=w448) -> (w446:i32[])
                  }
                  frame True {
                  }
                }
              }
            }
          }
          frame "TableWith2ndStrikerPlay" {
            n152 = property class="Playbook"(reference=w457) -> ("offensive_plays"=w453:T3)  [unwired: 1 in, 2 out]
            n153 = Unbundle By Name(w453) -> ("TableWith2ndStrikerPlay"=w451:refnum<class "TableWith2ndStrikerPlay.lvclass">)
            n154 = property class="Robot"(reference=w459) -> ("role"=w461:T4)  [unwired: 1 in, 2 out]
            n155 = property class="TablePlay"(reference=w451) -> ("Roles"=w452:T11)  [unwired: 1 in, 2 out]
            n156 = case shown="\"TableFinalizer\", Default" w461 {
              tunnel: w452 -> [w469 w488 w504]
              tunnel: w460 -> [w470 w481 w503]
              tunnel: [w465 w487 w502] -> w456
              tunnel: [w464 w483 w497] -> w455
              tunnel: w454 -> [w467 w482 w498]
              tunnel: w458 -> [w463 w479 w495]
              tunnel: w450 -> [w462 w478 w494]
              frame "PassObserver" {
                n157 = Unbundle By Name(w469) -> ("PassObserverRole"=w468:refnum<class "PassObserverRole.lvclass">)
                n158 = call "PassObserverRole.vi"("Tactic index in"=w462, "first call"=w463, "Game in"=w470, "PassObserverRole in"=w468) -> ("tactic index"=w466:i32, "Robot"=w465:refnum<class "Robot.lvclass">)  [unwired: 5 in, 1 out]
                n159 = Equal?(x=w466, y=-1) -> (x = y?=w471:bool)
                n160 = case shown="True" w471 {
                  tunnel: w466 -> [w476 _]
                  tunnel: w467 -> [w475 w477]
                  tunnel: [w474 w477] -> w464
                  frame False {
                    n161 = Insert Into Array(array=w475, index=0, new element=w476) -> (w474:i32[])
                  }
                  frame True {
                  }
                }
              }
              frame "TableFinalizer", Default {
                n162 = Unbundle By Name(w488) -> ("TableFinalizerRole"=w480:refnum<class "TableFinalizerRole.lvclass">)
                n163 = call "TableFinalizerRole.vi"("Tactic index in"=w478, "first call"=w479, "Game in"=w481, "TableFinalizerRole in"=w480) -> ("tactic index"=w484:i32, "Robot out"=w487:refnum<class "Robot.lvclass">)  [unwired: 4 in, 2 out]
                n164 = Equal?(x=w484, y=-1) -> (x = y?=w485:bool)
                n165 = case shown="True" w485 {
                  tunnel: w484 -> [w492 _]
                  tunnel: w482 -> [w491 w493]
                  tunnel: [w490 w493] -> w483
                  frame False {
                    n166 = Insert Into Array(array=w491, index=0, new element=w492) -> (w490:i32[])
                  }
                  frame True {
                  }
                }
              }
              frame "Tabler" {
                n167 = Unbundle By Name(w504) -> ("TablerRole"=w496:refnum<class "TablerRole.lvclass">)
                n168 = call "TablerRole.vi"("Tactic index in"=w494, "first call"=w495, "Game in"=w503, "TablerRole in"=w496) -> ("tactic index"=w499:i32, "Robot out"=w502:refnum<class "Robot.lvclass">)  [unwired: 4 in, 2 out]
                n169 = Equal?(x=w499, y=-1) -> (x = y?=w501:bool)
                n170 = case shown="False" w501 {
                  tunnel: w499 -> [w508 _]
                  tunnel: w498 -> [w507 w509]
                  tunnel: [w506 w509] -> w497
                  frame False {
                    n171 = Insert Into Array(array=w507, index=0, new element=w508) -> (w506:i32[])
                  }
                  frame True {
                  }
                }
              }
            }
          }
          frame "DirectEnemy" {
            n172 = property class="Playbook"(reference=w517) -> ("offensive_plays"=w516:T3)  [unwired: 1 in, 2 out]
            n173 = Unbundle By Name(w516) -> ("DirectEnemyPlay"=w515:refnum<class "DirectEnemyPlay.lvclass">)
            n174 = property class="Robot"(reference=w511) -> ("role"=w510:T4)  [unwired: 1 in, 2 out]
            n175 = property class="DirectEnemyPlay"(reference=w515) -> ("Roles"=w514:T12)  [unwired: 1 in, 2 out]
            n176 = case shown="\"Marker\"" w510 {
              tunnel: w514 -> [w521 w525]
              tunnel: w513 -> [w519 w523]
              tunnel: [w518 w522] -> w512
              frame "AttackerStop", Default {
                n177 = Unbundle By Name(w521) -> ("AttackerBlockRole"=w520:refnum<class "AttackerBlockRole.lvclass">)
                n178 = call-dynamic "AttackerBlockRole.vi"("Game in"=w519, "AttackerBlockRole in"=w520) -> ("Robot out"=w518:refnum<class "Robot.lvclass">)  [unwired: 6 in, 3 out]
              }
              frame "Marker" {
                n179 = Unbundle By Name(w525) -> ("MarkerRole"=w524:refnum<class "MarkerRole.lvclass">)
                n180 = call-dynamic "MarkerRole.vi"("Game in"=w523, "MarkerRole in"=w524) -> ("Robot out"=w522:refnum<class "Robot.lvclass">)  [unwired: 6 in, 3 out]
              }
            }
          }
          frame "Halt" {
            n181 = property class="Playbook"(reference=w533) -> ("offensive_plays"=w532:T3)  [unwired: 1 in, 2 out]
            n182 = Unbundle By Name(w532) -> ("HaltPlay"=w531:refnum<class "HaltPlay.lvclass">)
            n183 = property class="Robot"(reference=w527) -> ("role"=w526:T4)  [unwired: 1 in, 2 out]
            n184 = property class="HaltPlay"(reference=w531) -> ("Roles"=w530:T13)  [unwired: 1 in, 2 out]
            n185 = case shown="\"Halt\", Default" w526 {
              tunnel: w530 -> [w537]
              tunnel: w529 -> [w535]
              tunnel: [w534] -> w528
              frame "Halt", Default {
                n186 = Unbundle By Name(w537) -> ("HaltRole 1"=w536:refnum<class "HaltRole.lvclass">)
                n187 = call "HaltRole.vi"("Game in"=w535, "HaltRole in"=w536) -> ("Robot out"=w534:refnum<class "Robot.lvclass">)  [unwired: 6 in, 3 out]
              }
            }
          }
          frame "IndirectEnemy" {
            n188 = property class="Playbook"(reference=w545) -> ("offensive_plays"=w544:T3)  [unwired: 1 in, 2 out]
            n189 = Unbundle By Name(w544) -> ("IndirectEnemyPlay"=w543:refnum<class "IndirectEnemyPlay.lvclass">)
            n190 = property class="Robot"(reference=w539) -> ("role"=w538:T4)  [unwired: 1 in, 2 out]
            n191 = property class="IndirectEnemyPlay"(reference=w543) -> ("Roles"=w542:T12)  [unwired: 1 in, 2 out]
            n192 = case shown="\"AttackerBlock\", Default" w538 {
              tunnel: w542 -> [w549 w553]
              tunnel: w541 -> [w547 w551]
              tunnel: [w546 w550] -> w540
              frame "AttackerBlock", Default {
                n193 = Unbundle By Name(w549) -> ("AttackerBlockRole"=w548:refnum<class "AttackerBlockRole.lvclass">)
                n194 = call-dynamic "AttackerBlockRole.vi"("Game in"=w547, "AttackerBlockRole in"=w548) -> ("Robot out"=w546:refnum<class "Robot.lvclass">)  [unwired: 6 in, 3 out]
              }
              frame "Marker" {
                n195 = Unbundle By Name(w553) -> ("MarkerRole"=w552:refnum<class "MarkerRole.lvclass">)
                n196 = call-dynamic "MarkerRole.vi"("Game in"=w551, "MarkerRole in"=w552) -> ("Robot out"=w550:refnum<class "Robot.lvclass">)  [unwired: 6 in, 3 out]
              }
            }
          }
          frame "StopOffensive" {
            n197 = property class="Playbook"(reference=w561) -> ("offensive_plays"=w560:T3)  [unwired: 1 in, 2 out]
            n198 = Unbundle By Name(w560) -> ("StopOffensivePlay"=w559:refnum<class "StopOffensivePlay.lvclass">)
            n199 = property class="Robot"(reference=w554) -> ("role"=w555:T4)  [unwired: 1 in, 2 out]
            n200 = property class="StopOffensivePlay"(reference=w559) -> ("Roles"=w558:T14)  [unwired: 1 in, 2 out]
            n201 = case shown="\"AttackerStop\", Default" w555 {
              tunnel: w558 -> [w565 w569]
              tunnel: w557 -> [w564 w567]
              tunnel: [w563 w566] -> w556
              frame "AttackerStop", Default {
                n202 = Unbundle By Name(w565) -> ("AttackerStopRole"=w562:refnum<class "AttackerStopRole.lvclass">)
                n203 = call-dynamic "AttackerStopRole.vi"("Game in"=w564, "AttackerStopRole in"=w562) -> ("Robot out"=w563:refnum<class "Robot.lvclass">)  [unwired: 6 in, 3 out]
              }
              frame "Marker" {
                n204 = Unbundle By Name(w569) -> ("MarkerRole"=w568:refnum<class "MarkerRole.lvclass">)
                n205 = call-dynamic "MarkerRole.vi"("Game in"=w567, "MarkerRole in"=w568) -> ("Robot out"=w566:refnum<class "Robot.lvclass">)  [unwired: 6 in, 3 out]
              }
            }
          }
          frame "BallOutOfField" {
            n206 = property class="Playbook"(reference=w577) -> ("offensive_plays"=w576:T3)  [unwired: 1 in, 2 out]
            n207 = Unbundle By Name(w576) -> ("BallOutOfFieldPlay"=w575:refnum<class "BallOutOfFieldPlay.lvclass">)
            n208 = property class="Robot"(reference=w571) -> ("role"=w570:T4)  [unwired: 1 in, 2 out]
            n209 = property class="BallOutOfFieldPlay"(reference=w575) -> ("Roles"=w574:T15)  [unwired: 1 in, 2 out]
            n210 = case shown="\"BallOutOfField\", Default" w570 {
              tunnel: w574 -> [w581 w585]
              tunnel: w573 -> [w579 w583]
              tunnel: [w578 w582] -> w572
              frame "BallOutOfField", Default {
                n211 = Unbundle By Name(w581) -> ("BallOutOfFieldRole"=w580:refnum<class "BallOutOfFieldRole.lvclass">)
                n212 = call-dynamic "BallOutOfFieldRole.vi"("Game in"=w579, "BallOutOfFieldRole in"=w580) -> ("Robot out"=w578:refnum<class "Robot.lvclass">)  [unwired: 6 in, 3 out]
              }
              frame "FollowAttacker" {
                n213 = Unbundle By Name(w585) -> ("FollowAttackerRole"=w584:refnum<class "FollowAttackerRole.lvclass">)
                n214 = call "FollowAttackerRole.vi"("Game in"=w583, "FollowAttackerRole in"=w584) -> ("Robot out"=w582:refnum<class "Robot.lvclass">)  [unwired: 6 in, 3 out]
              }
            }
          }
          frame "EnemyPossessionAtEnemyField" {
            n215 = property class="Playbook"(reference=w593) -> ("offensive_plays"=w592:T3)  [unwired: 1 in, 2 out]
            n216 = Unbundle By Name(w592) -> ("EnemyPossessionAtEnemyFieldPlay"=w591:refnum<class "EnemyPossessionAtEnemyFieldPlay.lvclass">)
            n217 = property class="EnemyPossessionAtEnemyFieldPlay"(reference=w591) -> ("Roles"=w590:T16)  [unwired: 1 in, 2 out]
            n218 = property class="Robot"(reference=w587) -> ("role"=w586:T4)  [unwired: 1 in, 2 out]
            n219 = case shown="\"FollowAttacker\"" w586 {
              tunnel: w590 -> [w597 w601]
              tunnel: w589 -> [w596 w600]
              tunnel: [w594 w598] -> w588
              frame "Shoot", Default {
                n220 = Unbundle By Name(w597) -> ("ShootRole"=w595:refnum<class "ShootRole.lvclass">)
                n221 = call-dynamic "ShootRole.vi"("Game in"=w596, "ShootRole in"=w595) -> ("Robot out"=w594:refnum<class "Robot.lvclass">)  [unwired: 6 in, 3 out]
              }
              frame "FollowAttacker" {
                n222 = Unbundle By Name(w601) -> ("FollowAttackerRole"=w599:refnum<class "FollowAttackerRole.lvclass">)
                n223 = call "FollowAttackerRole.vi"("Game in"=w600, "FollowAttackerRole in"=w599) -> ("Robot out"=w598:refnum<class "Robot.lvclass">)  [unwired: 6 in, 3 out]
              }
            }
          }
          frame "NormalGame", "DirectKick", Default {
            n224 = property class="Playbook"(reference=w609) -> ("offensive_plays"=w608:T3)  [unwired: 1 in, 2 out]
            n225 = Unbundle By Name(w608) -> ("NormalGamePlay"=w607:refnum<class "NormalGamePlay.lvclass">)
            n226 = property class="Robot"(reference=w603) -> ("role"=w602:T4)  [unwired: 1 in, 2 out]
            n227 = property class="NormalGamePlay"(reference=w607) -> ("Roles"=w606:T16)  [unwired: 1 in, 2 out]
            n228 = case shown="\"FollowAttacker\"" w602 {
              tunnel: w606 -> [w613 w617]
              tunnel: w605 -> [w612 w616]
              tunnel: [w610 w614] -> w604
              frame "Shoot", Default {
                n229 = Unbundle By Name(w613) -> ("ShootRole"=w611:refnum<class "ShootRole.lvclass">)
                n230 = call-dynamic "ShootRole.vi"("Game in"=w612, "ShootRole in"=w611) -> ("Robot out"=w610:refnum<class "Robot.lvclass">)  [unwired: 6 in, 3 out]
              }
              frame "FollowAttacker" {
                n231 = Unbundle By Name(w617) -> ("FollowAttackerRole"=w615:refnum<class "FollowAttackerRole.lvclass">)
                n232 = call "FollowAttackerRole.vi"("Game in"=w616, "FollowAttackerRole in"=w615) -> ("Robot out"=w614:refnum<class "Robot.lvclass">)  [unwired: 6 in, 3 out]
              }
            }
          }
          frame "PrepareKickoffAlly" {
            n233 = property class="Playbook"(reference=w625) -> ("offensive_plays"=w624:T3)  [unwired: 1 in, 2 out]
            n234 = Unbundle By Name(w624) -> ("PrepareKickoffAllyPlay"=w623:refnum<class "PrepareKickoffAllyPlay.lvclass">)
            n235 = property class="Robot"(reference=w619) -> ("role"=w618:T4)  [unwired: 1 in, 2 out]
            n236 = property class="PrepareKickoffAllyPlay"(reference=w623) -> ("Roles"=w622:T17)  [unwired: 1 in, 2 out]
            n237 = case shown="\"AttackerAimGoal\", Default" w618 {
              tunnel: w622 -> [w629 w633]
              tunnel: w621 -> [w627 w632]
              tunnel: [w626 w630] -> w620
              frame "AttackerAimGoal", Default {
                n238 = Unbundle By Name(w629) -> ("AttackerAimGoalRole"=w628:refnum<class "AttackerAimGoalRole.lvclass">)
                n239 = call-dynamic "AttackerAimGoalRole.vi"("Game in"=w627, "AttackerAimGoalRole in"=w628) -> ("Robot out"=w626:refnum<class "Robot.lvclass">)  [unwired: 6 in, 3 out]
              }
              frame "FollowAttacker" {
                n240 = Unbundle By Name(w633) -> ("FollowAttackerRole"=w631:refnum<class "FollowAttackerRole.lvclass">)
                n241 = call "FollowAttackerRole.vi"("Game in"=w632, "FollowAttackerRole in"=w631) -> ("Robot out"=w630:refnum<class "Robot.lvclass">)  [unwired: 6 in, 3 out]
              }
            }
          }
          frame "PreparePenaltyAlly" {
            n242 = property class="Playbook"(reference=w641) -> ("offensive_plays"=w640:T3)  [unwired: 1 in, 2 out]
            n243 = Unbundle By Name(w640) -> ("PreparePenaltyAllyPlay"=w639:refnum<class "PreparePenaltyAllyPlay.lvclass">)
            n244 = property class="Robot"(reference=w635) -> ("role"=w634:T4)  [unwired: 1 in, 2 out]
            n245 = property class="PreparePenaltyAllyPlay"(reference=w639) -> ("Roles"=w638:T18)  [unwired: 1 in, 2 out]
            n246 = case shown="\"AttackerAimGoal\", Default" w634 {
              tunnel: w638 -> [w645]
              tunnel: w637 -> [w643]
              tunnel: [w642] -> w636
              frame "AttackerAimGoal", Default {
                n247 = Unbundle By Name(w645) -> ("AttackerAimGoalRole"=w644:refnum<class "AttackerAimGoalRole.lvclass">)
                n248 = call-dynamic "AttackerAimGoalRole.vi"("Game in"=w643, "AttackerAimGoalRole in"=w644) -> ("Robot out"=w642:refnum<class "Robot.lvclass">)  [unwired: 6 in, 3 out]
              }
            }
          }
          frame "Prepare Penalty Enemy" {
            n249 = property class="Playbook"(reference=w654) -> ("offensive_plays"=w653:T3)  [unwired: 1 in, 2 out]
            n250 = Unbundle By Name(w653) -> ("PreparePenaltyEnemyPlay"=w652:refnum<class "PreparePenaltyEnemyPlay.lvclass">)
            n251 = property class="Robot" props=["id"](reference=w649) -> ()  [unwired: 1 in, 3 out]
            n252 = property class="PreparePenaltyEnemyPlay"(reference=w652) -> ("roles"=w651:T19)  [unwired: 1 in, 2 out]
            n253 = Increment(x=w646) -> (x+1=w647:i32)
            n254 = case shown="5" w647 {
              tunnel: w651 -> [w658 w662 w666 w670 w674]
              tunnel: w650 -> [_ _ _ _ _]
              tunnel: [w656 w660 w664 w668 w672] -> w648
              tunnel: w646 -> [w655 w659 w663 w667 w671]
              frame 1, Default {
                n255 = Unbundle By Name(w658) -> ("PenaltyDefenseRole 1"=w657:refnum<class "PenaltyDefenseRole.lvclass">)
                n256 = call "PenaltyDefenseRole.vi"("IndexInVector"=w655, "PenaltyDefenseRole in"=w657) -> ("Robot out"=w656:refnum<class "Robot.lvclass">)  [unwired: 7 in, 2 out]
              }
              frame 2 {
                n257 = Unbundle By Name(w662) -> ("PenaltyDefenseRole 2"=w661:refnum<class "PenaltyDefenseRole.lvclass">)
                n258 = call "PenaltyDefenseRole.vi"("IndexInVector"=w659, "PenaltyDefenseRole in"=w661) -> ("Robot out"=w660:refnum<class "Robot.lvclass">)  [unwired: 7 in, 2 out]
              }
              frame 3 {
                n259 = Unbundle By Name(w666) -> ("PenaltyDefenseRole 3"=w665:refnum<class "PenaltyDefenseRole.lvclass">)
                n260 = call "PenaltyDefenseRole.vi"("IndexInVector"=w663, "PenaltyDefenseRole in"=w665) -> ("Robot out"=w664:refnum<class "Robot.lvclass">)  [unwired: 7 in, 2 out]
              }
              frame 4 {
                n261 = Unbundle By Name(w670) -> ("PenaltyDefenseRole 4"=w669:refnum<class "PenaltyDefenseRole.lvclass">)
                n262 = call "PenaltyDefenseRole.vi"("IndexInVector"=w667, "PenaltyDefenseRole in"=w669) -> ("Robot out"=w668:refnum<class "Robot.lvclass">)  [unwired: 7 in, 2 out]
              }
              frame 5 {
                n263 = Unbundle By Name(w674) -> ("PenaltyDefenseRole 5"=w673:refnum<class "PenaltyDefenseRole.lvclass">)
                n264 = call "PenaltyDefenseRole.vi"("IndexInVector"=w671, "PenaltyDefenseRole in"=w673) -> ("Robot out"=w672:refnum<class "Robot.lvclass">)  [unwired: 7 in, 2 out]
              }
            }
          }
          frame "SimplePass" {
            # "Aqui atribui a role\nSó colocar as roles"
            n265 = property class="Playbook"(reference=w680) -> ("offensive_plays"=w685:T3)  [unwired: 1 in, 2 out]
            n266 = Unbundle By Name(w685) -> ("SimplePassPlay"=w676:refnum<class "SimplePass.lvclass">)
            n267 = property class="Robot"(reference=w677) -> ("role"=w686:T4)  [unwired: 1 in, 2 out]
            n268 = property class="SimplePass"(reference=w676) -> ("Roles"=w675:T20)  [unwired: 1 in, 2 out]
            n269 = case shown="\"SimplePassRoll\", Default" w686 {
              tunnel: w675 -> [w694 w713]
              tunnel: w682 -> [w691 w703]
              tunnel: [w687 w705] -> w684
              tunnel: [w693 w709] -> w683
              tunnel: w678 -> [w695 w710]
              tunnel: w681 -> [w692 w708]
              tunnel: w679 -> [w689 w706]
              frame "SimplePassRoll", Default {
                n270 = Unbundle By Name(w694) -> ("SimplePassRollRole"=w690:refnum<class "SimplePassRollRole.lvclass">)
                n271 = call "SimplePassRollRole.vi"("Tactic index in"=w689, "first call"=w692, "Game in"=w691, "SimplePassRollRole in"=w690) -> ("tactic index"=w688:i32, "Robot out"=w687:refnum<class "Robot.lvclass">)  [unwired: 4 in, 2 out]
                n272 = Equal?(x=w688, y=-1) -> (x = y?=w696:bool)
                n273 = case shown="True" w696 {
                  tunnel: w688 -> [w701 _]
                  tunnel: w695 -> [w700 w702]
                  tunnel: [w699 w702] -> w693
                  frame False {
                    n274 = Insert Into Array(array=w700, index=0, new element=w701) -> (w699:i32[])
                  }
                  frame True {
                  }
                }
              }
              frame "SimplePassRollReceiver" {
                n275 = Unbundle By Name(w713) -> ("SimplePassReceiverRole"=w704:refnum<class "SimplePassReceiverRole.lvclass">)
                n276 = call "SimplePassReceiverRole.vi"("first call"=w708, "Game in"=w703, "Tactic index in"=w706, "SimplePassReceiverRole in"=w704) -> ("tactic index"=w707:i32, "Robot out"=w705:refnum<class "Robot.lvclass">)  [unwired: 4 in, 2 out]
                n277 = Equal?(x=w707, y=-1) -> (x = y?=w712:bool)
                n278 = case shown="True" w712 {
                  tunnel: w707 -> [w717 _]
                  tunnel: w710 -> [w716 w718]
                  tunnel: [w715 w718] -> w709
                  frame False {
                    n279 = Insert Into Array(array=w716, index=0, new element=w717) -> (w715:i32[])
                  }
                  frame True {
                  }
                }
              }
            }
          }
          frame "PrepareKickoffEnemy" {
            n280 = property class="Playbook"(reference=w726) -> ("offensive_plays"=w725:T3)  [unwired: 1 in, 2 out]
            n281 = Unbundle By Name(w725) -> ("PrepareKickoffEnemyPlay"=w724:refnum<class "PrepareKickoffEnemyPlay.lvclass">)
            n282 = property class="PrepareKickoffEnemyPlay"(reference=w724) -> ("Roles"=w723:T21)  [unwired: 1 in, 2 out]
            n283 = property class="Robot"(reference=w720) -> ("role"=w719:T4)  [unwired: 1 in, 2 out]
            n284 = case shown="\"AttackerBlock\", Default" w719 {
              tunnel: w723 -> [w730 w734]
              tunnel: w722 -> [w728 w733]
              tunnel: [w727 w731] -> w721
              frame "AttackerBlock", Default {
                n285 = Unbundle By Name(w730) -> ("AttackerBlockRole"=w729:refnum<class "AttackerBlockRole.lvclass">)
                n286 = call-dynamic "AttackerBlockRole.vi"("Game in"=w728, "AttackerBlockRole in"=w729) -> ("Robot out"=w727:refnum<class "Robot.lvclass">)  [unwired: 6 in, 3 out]
              }
              frame "FollowAttacker" {
                n287 = Unbundle By Name(w734) -> ("FollowAttackerRole"=w732:refnum<class "FollowAttackerRole.lvclass">)
                n288 = call "FollowAttackerRole.vi"("Game in"=w733, "FollowAttackerRole in"=w732) -> ("Robot out"=w731:refnum<class "Robot.lvclass">)  [unwired: 6 in, 3 out]
              }
            }
          }
          frame "KickPenaltyAlly" {
            n289 = property class="Playbook"(reference=w742) -> ("offensive_plays"=w741:T3)  [unwired: 1 in, 2 out]
            n290 = Unbundle By Name(w741) -> ("KickPenaltyAllyPlay"=w740:refnum<class "KickPenaltyAllyPlay.lvclass">)
            n291 = property class="Robot"(reference=w736) -> ("role"=w735:T4)  [unwired: 1 in, 2 out]
            n292 = property class="KickPenaltyAllyPlay"(reference=w740) -> ("Roles"=w739:T22)  [unwired: 1 in, 2 out]
            n293 = case shown="\"PenaltyAttacker\", Default" w735 {
              tunnel: w739 -> [w746]
              tunnel: w738 -> [w744]
              tunnel: [w743] -> w737
              frame "PenaltyAttacker", Default {
                n294 = Unbundle By Name(w746) -> ("PenaltyAttackerRole"=w745:refnum<class "PenaltyAttackerRole.lvclass">)
                n295 = call "PenaltyAttackerRole.vi"("Game in"=w744, "PenaltyAttackerRole in"=w745) -> ("Robot out"=w743:refnum<class "Robot.lvclass">)  [unwired: 7 in, 2 out]
              }
            }
          }
        }
      }
      n296 = call-dynamic "findMinimumValueInArray.vi"("array"=w12, "Utilities in"=refnum<class "Utilities.lvclass"> refnum) -> ("minimum"=w20:dbl)  [unwired: 7 in, 2 out]
      n297 = feedback-in #2(w20) -> ()
      n298 = Empty Array?(array=w12) -> (empty?=w13:bool)
      n299 = property class="Ally"(reference=w7, "RobotRef"=w6, "OffensivePlay Finished"=w13, "StrikerPositioned_"=w10, "2ndStrikerPositioned_"=w10) -> (reference out=w22:refnum<class "Ally.lvclass">)  [unwired: 1 in, 1 out]
      n300 = property class="Game"(reference=w8, "OffensiveTeam"=w22) -> (reference out=w23:refnum<class "Game.lvclass">)  [unwired: 1 in, 1 out]
    }
    frame Error {
    }
  }
  "error out" <- w1
  "Game out" <- w2
